vi "Dio3216.vi"(7 "DIO3216B_Action":T2, 8 "Error in":errorcluster, 11 "IO In":T1 {"Port" items=["Input Port #1", "Input Port #2", "Out Port #1", "Out Port #2"]}) -> (0 "Error Out":errorcluster, 3 "IO Out":T1 {"Port" items=["Input Port #1", "Input Port #2", "Out Port #1", "Out Port #2"]})   [LabVIEW 2015]
uses:
  Main_IO #.ctl
  Dio3216_controls.ctl
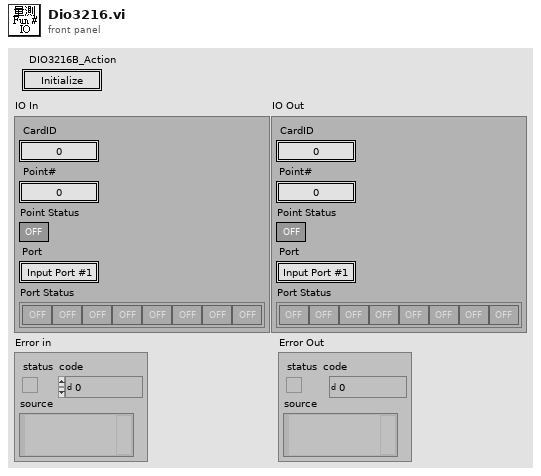
[diagram p1: front panel]
types:
  T1 = typedef "Main_IO #.ctl" = cluster{"CardID":u8, "Point#":u8, "Point Status":bool, "Port":u8, "Port Status":bool[]}
  T2 = typedef "Dio3216_controls.ctl" = enum16{"Initialize", "Set Point", "Set Port", "Read In Point", "Read Out Point", "Read Port", "Close", "Idle"}
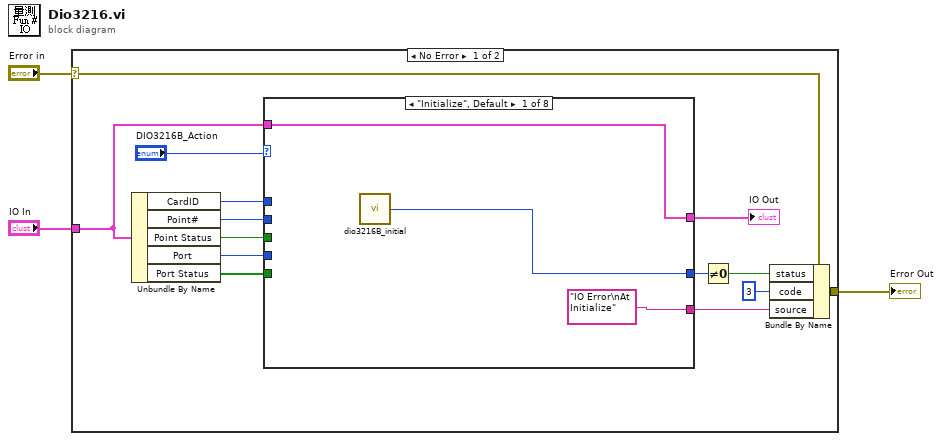
[diagram p0: block diagram]
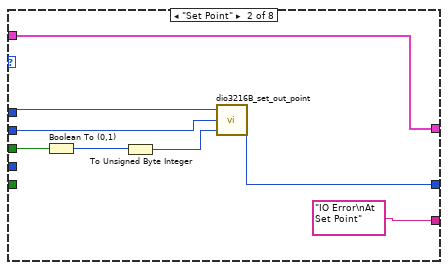
[diagram p2: hidden frame]
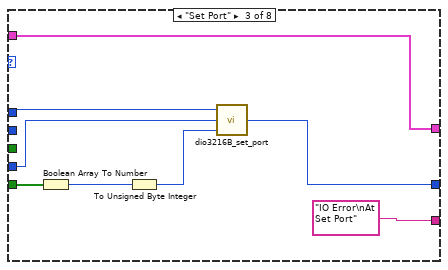
[diagram p3: hidden frame]
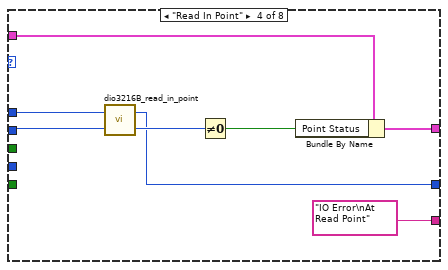
[diagram p4: hidden frame]
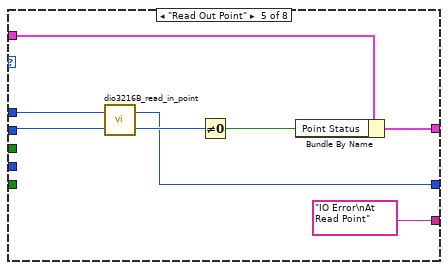
[diagram p5: hidden frame]
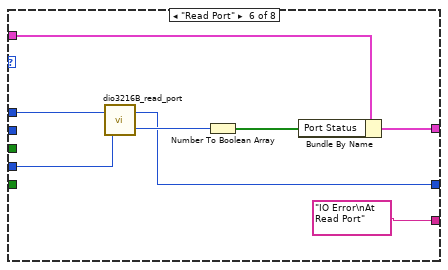
[diagram p6: hidden frame]
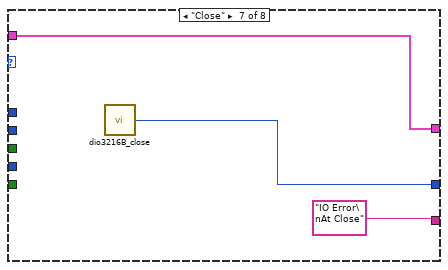
[diagram p7: hidden frame]
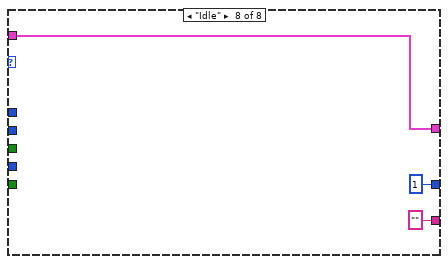
[diagram p8: hidden frame]
diagram:
  n1 = case shown="No Error" "Error in" {
    selector: "Error in" -> [w6 w67]
    tunnel: "IO In" -> [w12 _]
    tunnel: [w10 w67] -> w2
    frame No Error {
      n2 = Unbundle By Name(w12) -> ("CardID"=w17:u8, "Point#"=w16:u8, "Point Status"=w14:bool, "Port"=w15:u8, "Port Status"=w13:bool[])
      n3 = case shown="\"Initialize\", Default" "DIO3216B_Action" {
        tunnel: w17 -> [_ w28 w36 w44 w50 w60 _ _]
        tunnel: w16 -> [_ w27 _ w43 w49 _ _ _]
        tunnel: w14 -> [_ w26 _ _ _ _ _ _]
        tunnel: w15 -> [_ _ w35 _ _ w59 _ _]
        tunnel: w13 -> [_ _ w34 _ _ _ _ _]
        tunnel: w12 -> [w20 w23 w31 w42 w48 w56 w63 w66]
        tunnel: [w20 w23 w31 w41 w47 w57 w63 w66] -> w5
        tunnel: [w19 w22 w30 w38 w46 w54 w62 u32 1 ("error_code")] -> w11
        tunnel: ["IO Error\nAt Initialize" "IO Error\nAt Set Point" "IO Error\nAt Set Port" "IO Error\nAt Read Point" "IO Error\nAt Read Point" "IO Error\nAt Read Port" "IO Error\nAt Close" ""] -> w7
        frame "Initialize", Default {
          n4 = call <vilib>:"dio3216B_initial.vi"() -> ("error_code"=w19:u32)
        }
        frame "Set Point" {
          n5 = Boolean To (0,1)(Boolean=w26) -> (0, 1=w25:i16)
          n6 = To Unsigned Byte Integer(number=w25) -> (unsigned 8bit integer=w24:u8)
          n7 = call <vilib>:"dio3216B_set_out_point.vi"("state"=w24, "point"=w27, "CardID"=w28) -> ("error_code"=w22:u32)
        }
        frame "Set Port" {
          n8 = Boolean Array To Number(Boolean array=w34) -> (number=w33:u32)
          n9 = To Unsigned Byte Integer(number=w33) -> (unsigned 8bit integer=w32:u8)
          n10 = call <vilib>:"dio3216B_set_port.vi"("data"=w32, "port"=w35, "CardID"=w36) -> ("error_code"=w30:u32)
        }
        frame "Read In Point" {
          n11 = call <vilib>:"dio3216B_read_in_point.vi"("point"=w43, "CardID"=w44) -> ("state"=w40:u8, "error_code"=w38:u32)
          n12 = Not Equal To 0?(x=w40) -> (x != 0?=w39:bool)
          n13 = Bundle By Name(cluster=w42, "Point Status"=w39) -> (w41:T1)
        }
        frame "Read Out Point" {
          n14 = call <vilib>:"dio3216B_read_in_point.vi"("point"=w49, "CardID"=w50) -> ("state"=w52:u8, "error_code"=w46:u32)
          n15 = Not Equal To 0?(x=w52) -> (x != 0?=w51:bool)
          n16 = Bundle By Name(cluster=w48, "Point Status"=w51) -> (w47:T1)
        }
        frame "Read Port" {
          n17 = call <vilib>:"dio3216B_read_port.vi"("port"=w59, "CardID"=w60) -> ("data"=w58:u8, "error_code"=w54:u32)
          n18 = Number To Boolean Array(number=w58) -> (Boolean array=w55:bool[])
          n19 = Bundle By Name(cluster=w56, "Port Status"=w55) -> (w57:T1)
        }
        frame "Close" {
          n20 = call <vilib>:"dio3216B_close.vi"() -> ("error_code"=w62:u32)
        }
        frame "Idle" {
        }
      }
      "IO Out" <- w5
      n21 = Not Equal To 0?(x=w11) -> (x != 0?=w9:bool)
      n22 = Bundle By Name(cluster=w6, "status"=w9, "code"=3, "source"=w7) -> (w10:errorcluster)
    }
    frame Error {
    }
  }
  "Error Out" <- w2
